vi "Perform Action.vi"(8 "error in (no error)":errorcluster, 10 "Input":variant, 11 "Virt Instrument Base in":refnum<class "Virt Temperature Reader.lvclass">) -> (0 "error out":errorcluster, 2 "Output":variant, 3 "Virt Instrument Base out":refnum<class "Virt Temperature Reader.lvclass">)   [LabVIEW 2023, in "Virt Instrs Thermometer.lvlib" / "Virt Temperature Reader.lvclass"]
uses:
  Virt Temperature Reader.lvclass
  Virt Temperature Reader.lvclass/Virt Temperature Reader.ctl
  <vilib>/Analysis/NI_AALBase.lvlib
  <vilib>/Analysis/baseanly.llb/Mean (DBL).vi
  Virtual Instrument Base/Virt Instr Base.lvclass
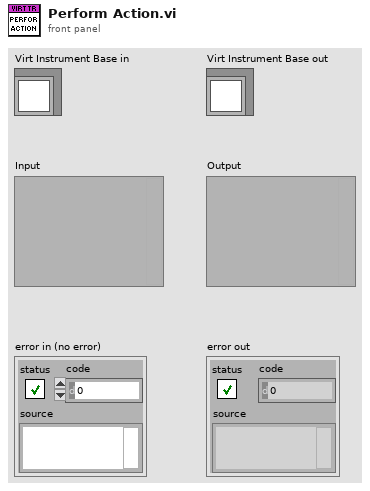
[diagram p1: front panel]
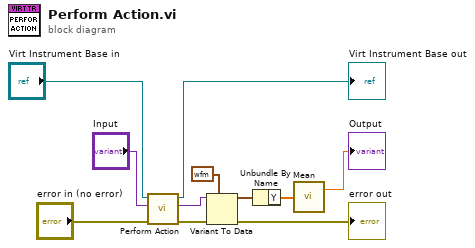
[diagram p0: block diagram]
diagram:
  n1 = call-parent "Perform Action.vi"("error in (no error)"="error in (no error)", "Input"="Input", "Virt Instrument Base in"="Virt Instrument Base in") -> ("error out"=w4:errorcluster, "Output"=w3:variant, "Virt Instrument Base out"=→"Virt Instrument Base out":refnum<class "Virt Temperature Reader.lvclass">)  [unwired: 6 in]
  n2 = Variant To Data(error in=w4, type=waveform(dbl) {"t0"=timestamp(0 s since 1904-01-01), "dt"=1.0, "Y"=[]} ("Waveform"), Variant=w3) -> (data=w7:waveform(dbl), error out=→"error out":errorcluster)
  n3 = Unbundle By Name(w7) -> ("Y"=w5:dbl[])
  n4 = call-poly <vilib>:"Mean.vi"("X"=w5) -> ("mean"=→"Output":dbl)  [unwired: 1 out]
